vi "testCreateTcpServer.vi"(8 "error in (no error)":errorcluster) -> (0 "error out":errorcluster)   [LabVIEW 2018]
uses:
  src/FactoryTcpServer/FactoryTcpServer.lvclass
  <vilib>/addons/_JKI Toolkits/Caraya/classes/Test/Test.lvclass
  <vilib>/addons/_JKI Toolkits/Caraya/classes/Assert/Assert.lvclass
  <vilib>/addons/_JKI Toolkits/Caraya/classes/Assert/Assert Equal Value_Variant.vi
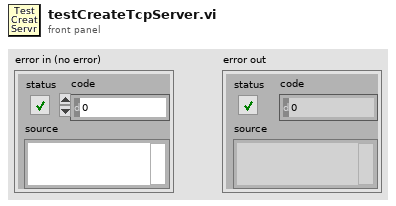
[diagram p1: front panel]
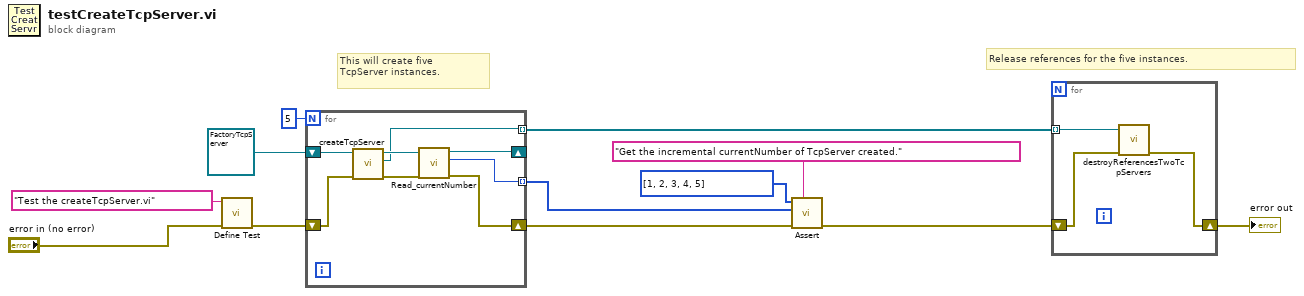
[diagram p0: block diagram]
diagram:
  # "Release references for the five instances."
  # "This will create five \nTcpServer instances."
  n1 = call <vilib>:"Define Test.vi"("error in (no error)"="error in (no error)", "Label (VI Title)"="Test the createTcpServer.vi") -> ("error out"=w9:errorcluster)  [unwired: 9 in]
  n2 = for {
    N: 5 -> [_]
    shift-right: [w17] -> _
    shift-left: refnum<class "FactoryTcpServer.lvclass"> refnum ("FactoryTcpServer.lvclass") -> [w20]
    tunnel: [w16] -> w4 mode=indexing
    shift-right: [w15] -> w6
    shift-left: w9 -> [w14]
    tunnel: [w13] -> w1 mode=indexing
    n3 = call "createTcpServer.vi"("error in (no error)"=w14, "FactoryTcpServer in"=w20) -> ("error out"=w18:errorcluster, "TcpServer out"=w13:refnum<class "TcpServer.lvclass">, "FactoryTcpServer out"=w19:refnum<class "FactoryTcpServer.lvclass">)  [unwired: 7 in]
    n4 = call "Read_currentNumber.vi"("error in (no error)"=w18, "FactoryTcpServer in"=w19) -> ("error out"=w15:errorcluster, "currentNumber"=w16:i32, "FactoryTcpServer out"=w17:refnum<class "FactoryTcpServer.lvclass">)  [unwired: 7 in]
  }
  n5 = call-poly <vilib>:"Assert.vi"("Label"="Get the incremental currentNumber of TcpServer created.", "error in (no error)"=w6, "Y"=w4, "X"=i32[] [1, 2, 3, 4, 5] ("Array")) -> ("error out"=w3:errorcluster)  [unwired: 7 in]
  n6 = for {
    shift-right: [w21] -> w2
    shift-left: w3 -> [w22]
    tunnel: w1 -> [w23] mode=indexing
    n7 = call "destroyReferencesTwoTcpServers.vi"("error in (no error)"=w22, "TcpServer in"=w23) -> ("error out"=w21:errorcluster)  [unwired: 8 in, 1 out]
  }
  "error out" <- w2
